vi "Calculate Load.vi"(8 "error in (no error)":errorcluster, 11 "Proto in":refnum<class "Board.lvclass">) -> (0 "error out":errorcluster, 2 "Load":u64, 3 "Proto out":refnum<class "Board.lvclass">)   [LabVIEW 2021, in "Board.lvclass"]
uses:
  Board.lvclass
  Board.lvclass/Board.ctl
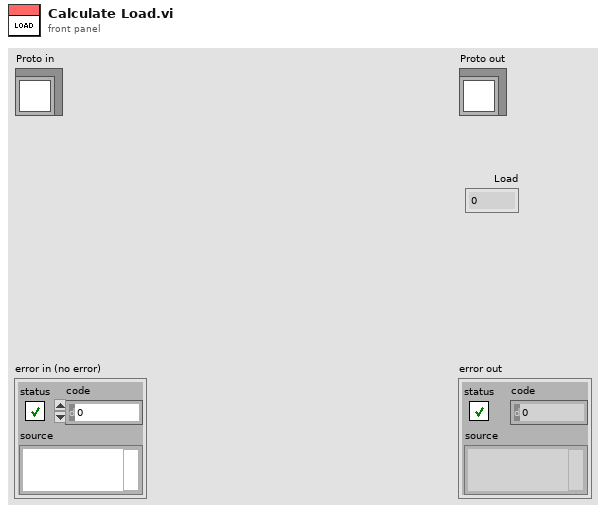
[diagram p1: front panel]
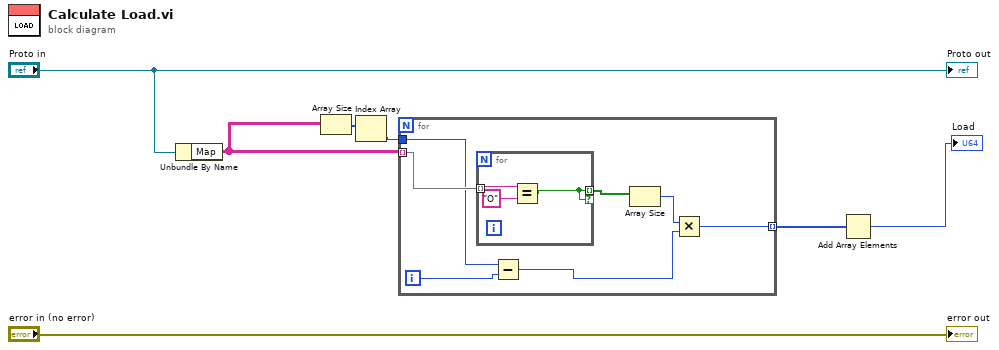
[diagram p0: block diagram]
diagram:
  n1 = Unbundle By Name("Proto in") -> ("Map"=w5:string[][])
  n2 = Array Size(array=w5) -> (size(s)=w2:i32[])
  n3 = Index Array(array=w2) -> (element=w1:i32)  [unwired: 1 in]
  n4 = for {
    tunnel: w5 -> [w11] mode=indexing
    tunnel: [w12] -> w3 mode=indexing
    tunnel: w1 -> [w10]
    i -> [w9]
    n5 = for {
      tunnel: w11 -> [w17] mode=indexing
      tunnel: [w15] -> w14 mode=indexing if=w15
      n6 = Equal?(x=w17, y="O") -> (x = y?=w15:bool)
    }
    n7 = Subtract(x=w10, y=w9) -> (x-y=w8:i32)
    n8 = Array Size(array=w14) -> (size(s)=w13:i32)
    n9 = Multiply(x=w13, y=w8) -> (x*y=w12:i32)
  }
  n10 = Add Array Elements(numeric array=w3) -> (sum=→"Load":i32)
  "error out" <- "error in (no error)"
  "Proto out" <- "Proto in"
